vi "sonde data collection.vi"() -> ()   [LabVIEW 2016]
uses:
  Groundwater header.ctl
  sample data row cluster.ctl
  sonde cluster.ctl
  <vilib>/Utility/NIReport.llb/NI_report.lvclass
panel:
  out "Current Sample Sheet":string
  in  "stop":bool
  out "row max value":i32
  in  "Write Data Line":bool
  out "last occupied cell's name":string
  in  "Final Data for Sample Sheet?":bool
  in  "Sample Sheet Data Row Cluster":T1={"Head"=0.0, "Depth"=0.0, "comment string"="", "Sonde Data Cluster"={"Cumulative\nVolume"=100.0, "Specific\nConductance"=2.0, "Dissolved\nOxygen"=3.0, "pH"=4.0, "ORP"=5.0, "Temp"=26.0, "Salinity"=7.0}} {"Sonde Data Cluster"."Salinity" format="%_3g"; "Sonde Data Cluster"."Temp" format="%_2g"; "Sonde Data Cluster"."ORP" format="%_4g"; "Sonde Data Cluster"."pH" format="%_4g"; "Sonde Data Cluster"."Dissolved\nOxygen" format="%_4g"; "Sonde Data Cluster"."Specific\nConductance" format="%_4g"; "Sonde Data Cluster"."Cumulative\nVolume" format="%#_4g"}
  out "number of rows":i32
  in  "report file path 2":path=path "D:/Cascade/templates/Groundwater Profiling Log_empty_2.xlsx"
  out "data":string[][](array[string])
  out "Elapsed Time (ms)":u32
  in  "error in (no error)":errorcluster
  in  "Groundwater Header":T3
  out "Worksheet Names":string[](array[string])
  in  "template file path":path=path "D:/Cascade/templates/Groundwater Profiling Log_empty_labview_template.xlsx"
  out "error out":errorcluster
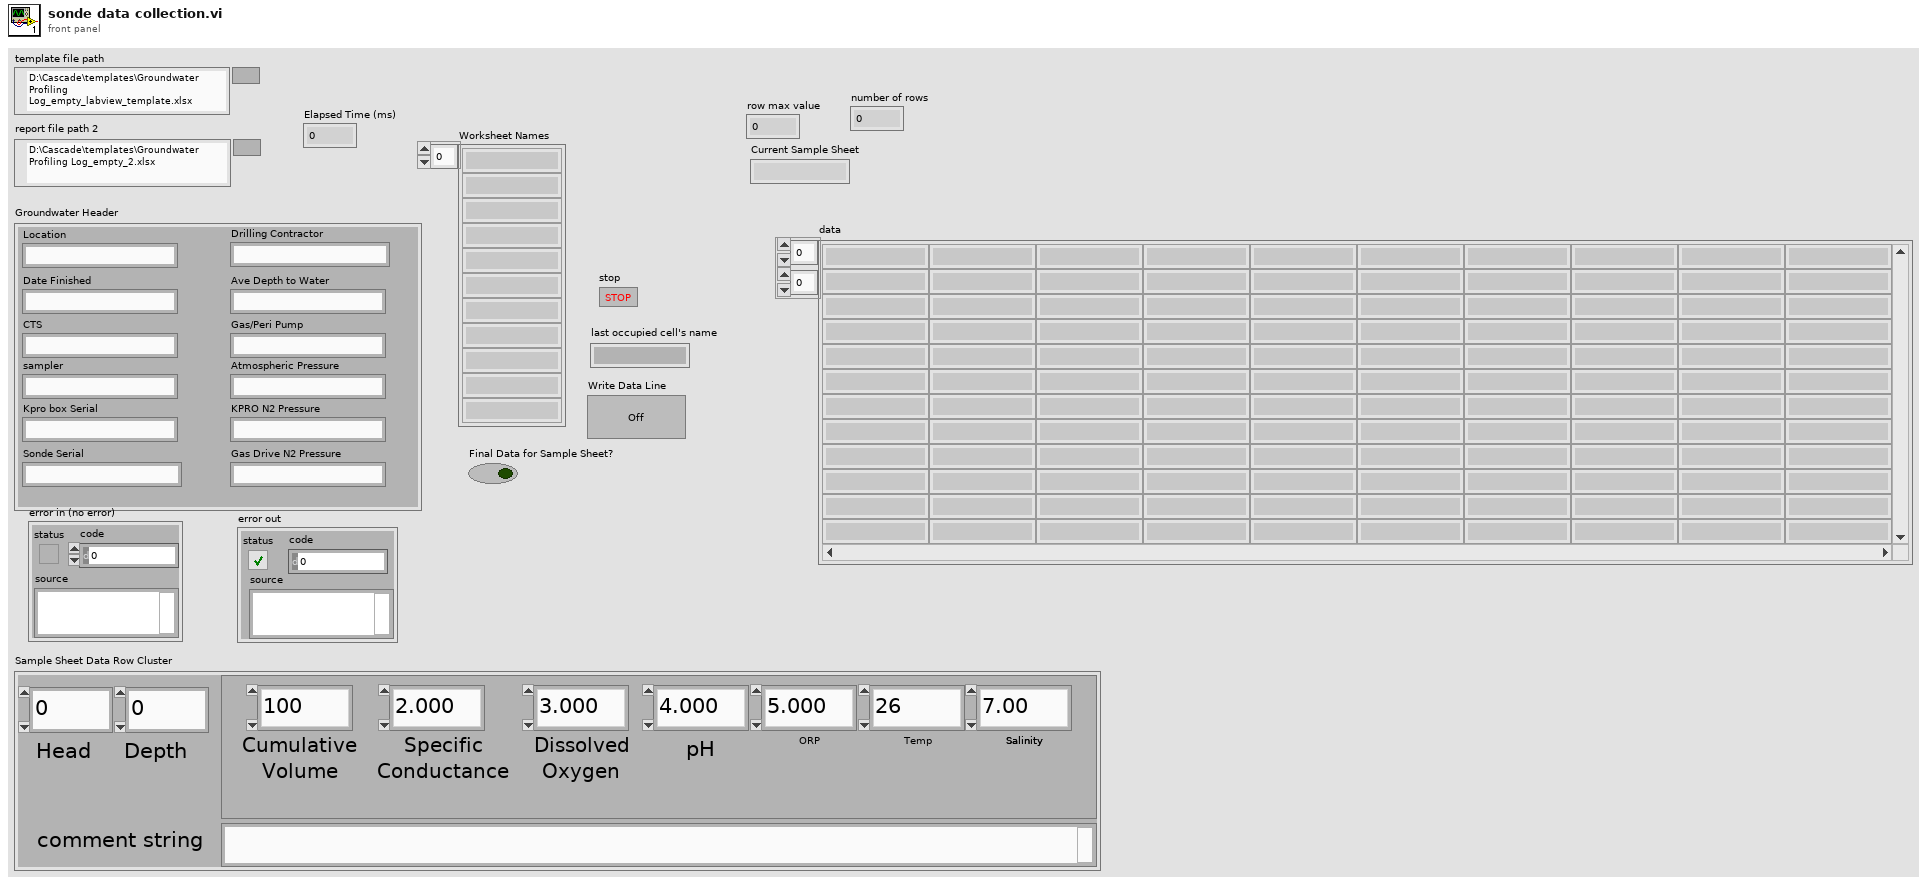
[diagram p1: front panel]
types:
  T1 = typedef "sample data row cluster.ctl" = cluster{"Head":dbl, "Depth":dbl, "comment string":string, "Sonde Data Cluster":T2}
  T2 = typedef "sonde cluster.ctl" = cluster{"Cumulative\nVolume":dbl, "Specific\nConductance":dbl, "Dissolved\nOxygen":dbl, "pH":dbl, "ORP":dbl, "Temp":dbl, "Salinity":dbl}
  T3 = typedef "Groundwater header.ctl" = cluster{"Location":string, "Date Finished":string, "CTS":string, "sampler":string, "Kpro box Serial ":string, "Sonde Serial":string, "Drilling Contractor":string, "Ave Depth to Water":string, "Gas/Peri Pump":string, "Atmospheric Pressure":string, "KPRO N2 Pressure":string, "Gas Drive N2 Pressure":string}
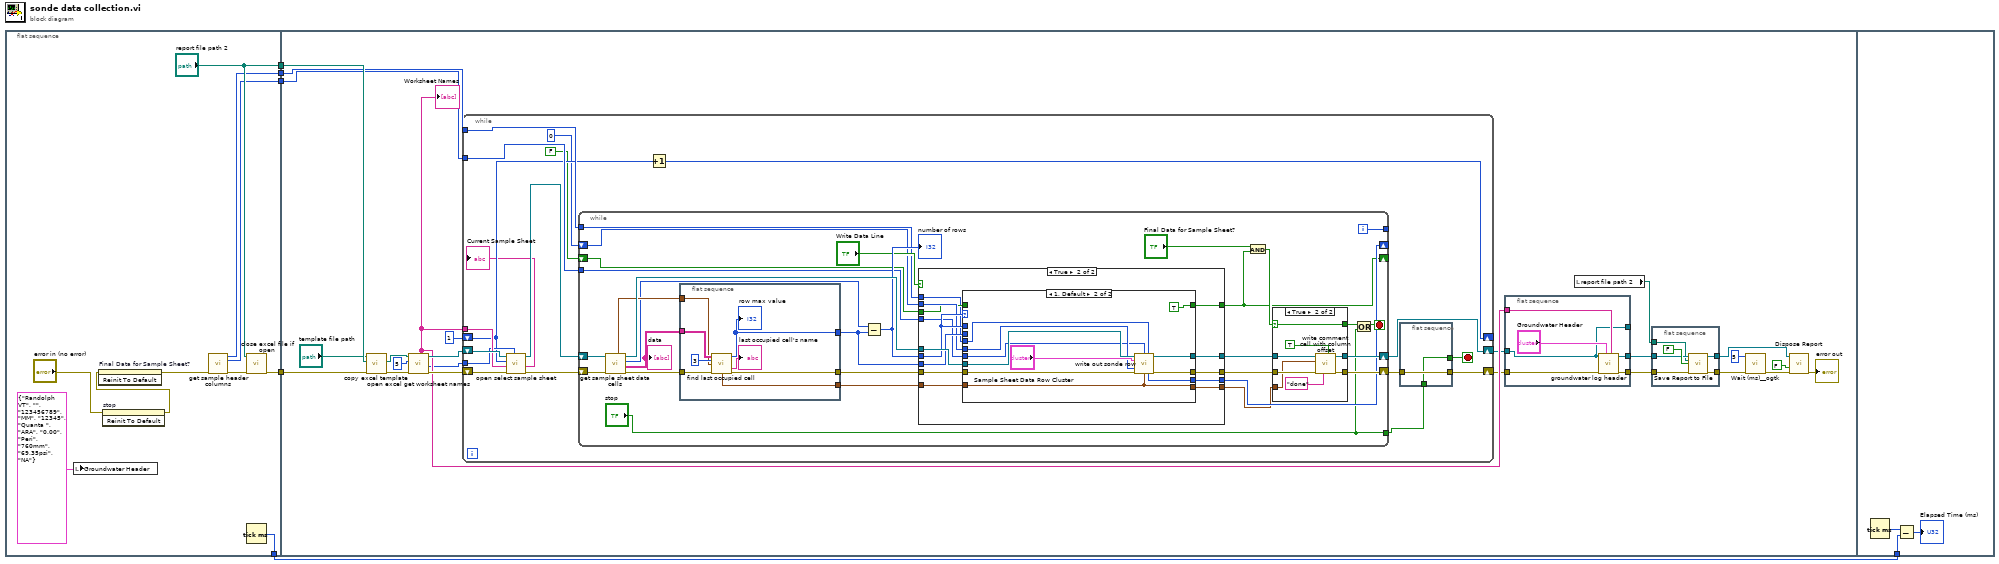
[diagram p0: block diagram]
diagram:
  n1 = flat-sequence {
    tunnel: [w14] -> w5
    tunnel: [w12] -> w4
    tunnel: ["report file path 2"] -> w3
    tunnel: [w10] -> w2
    tunnel: [w9] -> w1
    tunnel: w4 -> [w26]
    tunnel: w3 -> [w24]
    tunnel: w2 -> [w19]
    tunnel: w1 -> [w18]
    tunnel: w5 -> [w156]
    frame #0 {
      n2 = local write "Groundwater Header"(T3 {"Location"="Randolph VT", "Date Finished"="", "CTS"="123456789", "sampler"="MM", "Kpro box Serial "="12345", "Sonde Serial"="Quanta ", "Drilling Contractor"="ARA", "Ave Depth to Water"="0.00", "Gas/Peri Pump"="Peri", "Atmospheric Pressure"="760mm", "KPRO N2 Pressure"="69.35psi", "Gas Drive N2 Pressure"="NA"} ("Groundwater Header 2")) -> ()
      n3 = invoke on="stop" class="Bool" method="Reinit To Default"(error in="error in (no error)") -> (error out=w6:errorcluster)  [unwired: 2 in, 2 out]
      n4 = invoke on="Final Data for Sample Sheet?" class="Bool" method="Reinit To Default"(error in=w6) -> (error out=w11:errorcluster)  [unwired: 2 in, 2 out]
      n5 = call "get sample header columns.vi"("error in (no error)"=w11) -> ("Column of Volume"=w10:i32, "Columns"=w9:i32[], "error out"=w8:errorcluster)  [unwired: 5 in, 7 out]
      n6 = call "close excel file if open.vi"("error in (no error)"=w8, "report file path in"="report file path 2") -> ("error out"=w12:errorcluster)  [unwired: 8 in, 1 out]
      n7 = Tick Count (ms)() -> (millisecond timer value=w14:u32)
    }
    frame #1 {
      n8 = call "copy excel template.vi"("error in (no error)"=w26, "report file path in"=w24, "template file path in"="template file path") -> ("error out"=w22:errorcluster, "report file path out"=w25:path)  [unwired: 7 in]
      n9 = call "open excel get worksheet names.vi"("error in (no error)"=w22, "milliseconds to wait"=u32 5, "report file path"=w25) -> ("error out"=w32:errorcluster, "Number of Sample Sheets"=w17:i32, "NI_report out"=w31:refnum<class "NI_report.lvclass">, "Worksheet Names"=w29:string[])  [unwired: 3 in, 2 out]
      "Worksheet Names" <- w29
      n10 = while {
        tunnel: w29 -> [w54]
        tunnel: w19 -> [w51]
        tunnel: w18 -> [w50]
        tunnel: w17 -> [w49]
        shift-right: [w43] -> w21
        shift-left: w32 -> [w56]
        shift-right: [w52] -> w20
        shift-left: w31 -> [w55]
        shift-right: [w46] -> _
        shift-left: 1 ("input 1") -> [w47]
        stop <- w48 stop-if-true
        n11 = call "open select sample sheet.vi"("Number of Sample Sheets"=w49, "error in (no error)"=w56, "Worksheet Names"=w54, "input 1"=w47, "NI_report in"=w55) -> ("error out"=w53:errorcluster, "Current Sample Sheet"=→"Current Sample Sheet":string, "NI_report out"=w57:refnum<class "NI_report.lvclass">)  [unwired: 4 in]
        n12 = while {
          shift-right: [w73] -> w52
          shift-left: w57 -> [w86]
          shift-right: [w75] -> w44
          shift-left: w53 -> [w77]
          tunnel: [w70] -> _
          shift-right: [w68] -> _
          shift-left: 0 ("row index") -> [w69]
          shift-right: [w62] -> _
          shift-left: FALSE ("x") -> [w65]
          tunnel: w51 -> [w64]
          tunnel: w50 -> [w63]
          tunnel: ["stop"] -> w42
          i -> [w70]
          stop <- w59 stop-if-true
          n13 = call "get sample sheet data cells.vi"("error in (no error)"=w77, "NI_report in"=w86) -> ("error out"=w84:errorcluster, "data"=w78:string[][], "row"=w82:i32, "NI_report out"=w85:refnum<class "NI_report.lvclass">, "output cluster"=w83:cluster{"row":i32, "column":i32})  [unwired: 5 in]
          "data" <- w78
          n14 = flat-sequence {
            tunnel: w84 -> [w140]
            tunnel: w78 -> [w139]
            tunnel: w83 -> [w137]
            tunnel: [w136] -> w80
            tunnel: [w135] -> w79
            tunnel: [w134] -> w72
            frame #0 {
              n15 = call "find last occupied cell.vi"("data"=w139, "Header Rows to remove"=3, "sub array start"=w137, "error in (no error)"=w140) -> ("row max value"=w135:i32, "last occupied cell's name"=→"last occupied cell's name":string, "start of last occupied row"=w134:cluster{"row":i32, "column":i32}, "error out"=w136:errorcluster)  [unwired: 5 in, 3 out]
              "row max value" <- w135
            }
          }
          n16 = Subtract(x=w82, y=w79) -> (x-y=w81:i32)
          "number of rows" <- w81
          n17 = case shown="True" "Write Data Line" {
            tunnel: w85 -> [w91 w105]
            tunnel: w81 -> [_ w104]
            tunnel: w80 -> [w90 w103]
            tunnel: w79 -> [_ w102]
            tunnel: [w90 w101] -> w76
            tunnel: [w91 w100] -> w74
            tunnel: w72 -> [w88 w99]
            tunnel: w69 -> [w89 w98]
            tunnel: [w89 w97] -> w68
            tunnel: [w88 w96] -> w66
            tunnel: w65 -> [w87 w95]
            tunnel: [w87 w94] -> w62
            tunnel: w64 -> [_ w93]
            tunnel: w63 -> [_ w92]
            frame False {
            }
            frame True {
              n18 = case shown="1, Default" w104 {
                tunnel: [w109 w120] -> w101
                tunnel: [w110 w121] -> w100
                tunnel: w105 -> [w110 w119]
                tunnel: w99 -> [w107 w116]
                tunnel: w104 -> [_ _]
                tunnel: w103 -> [w109 w113]
                tunnel: w102 -> [_ _]
                tunnel: w98 -> [w108 w117]
                tunnel: [w108 w114] -> w97
                tunnel: [w107 w116] -> w96
                tunnel: w95 -> [w106 _]
                tunnel: [w106 TRUE ("x")] -> w94
                tunnel: w93 -> [_ w112]
                tunnel: w92 -> [_ w111]
                frame 0 {
                }
                frame 1, Default {
                  n19 = call "write out sonde row.vi"("NI_report in"=w119, "Columns"=w111, "Column of Volume"=w112, "Sample Sheet Data Row Cluster"="Sample Sheet Data Row Cluster", "row index"=w117, "error in (no error)"=w113, "start of last occupied row"=w116) -> ("NI_report out"=w121:refnum<class "NI_report.lvclass">, "row index out"=w114:i32, "error out"=w120:errorcluster)  [unwired: 6 in]
                }
              }
            }
          }
          n20 = And(x="Final Data for Sample Sheet?", y=w62) -> (x .and. y?=w67:bool)
          n21 = case shown="True" w67 {
            selector: w67 -> [w122 w125]
            tunnel: w76 -> [w123 w132]
            tunnel: [w123 w131] -> w75
            tunnel: w74 -> [w124 w130]
            tunnel: [w124 w129] -> w73
            tunnel: w66 -> [_ w127]
            tunnel: [w122 w125] -> w60
            frame False {
            }
            frame True {
              n22 = call "write comment cell with column offset.vi"("Column Relative?"=TRUE, "comment string"="done", "error in (no error)"=w132, "start of last occupied row"=w127, "NI_report in"=w130) -> ("error out"=w131:errorcluster, "NI_report out"=w129:refnum<class "NI_report.lvclass">)  [unwired: 5 in]
            }
          }
          n23 = Or(x=w60, y="stop") -> (x .or. y?=w59:bool)
        }
        n24 = Increment(x=w47) -> (x+1=w46:i32)
        n25 = flat-sequence {
          tunnel: [w141] -> w48
          tunnel: w44 -> [w142]
          tunnel: [w142] -> w43
          tunnel: w42 -> [w141]
          frame #0 {
          }
        }
      }
      n26 = flat-sequence {
        tunnel: w21 -> [w147]
        tunnel: [w146] -> w28
        tunnel: [w143] -> _
        tunnel: [w145] -> w30
        tunnel: w29 -> [w144]
        tunnel: w20 -> [w143]
        frame #0 {
          n27 = call "groundwater log header.vi"("Worksheet Names"=w144, "Groundwater Header"="Groundwater Header", "error in (no error)"=w147, "NI_report in"=w143) -> ("error out"=w146:errorcluster, "NI_report out"=w145:refnum<class "NI_report.lvclass">)  [unwired: 6 in]
        }
      }
      n28 = local read "report file path 2"() -> (w27:path)
      n29 = flat-sequence {
        tunnel: [w154] -> w39
        tunnel: [w153] -> w38
        tunnel: w28 -> [w151]
        tunnel: w30 -> [w150]
        tunnel: w27 -> [w149]
        frame #0 {
          n30 = call-dynamic "Save Report to File.vi"("report in"=w150, "report file path"=w149, "prompt to replace? (F)"=FALSE, "error in (no error)"=w151) -> ("report out"=w154:refnum<class "NI_report.lvclass">, "error out"=w153:errorcluster)  [unwired: 10 in]
        }
      }
      n31 = call <userlib>:"Wait (ms)__ogtk.vi"("error in (no error)"=w38, "milliseconds to wait"=u32 5) -> ("error out"=w35:errorcluster)  [unwired: 8 in, 1 out]
      n32 = call-dynamic "Dispose Report.vi"("report in"=w39, "save changes? (F)"=FALSE, "error in (no error)"=w35) -> ("error out"=→"error out":errorcluster)  [unwired: 12 in]
    }
    frame #2 {
      n33 = Tick Count (ms)() -> (millisecond timer value=w157:u32)
      n34 = Subtract(x=w157, y=w156) -> (x-y=→"Elapsed Time (ms)":u32)
    }
  }
